vi "Pre-Build Action.vi"(6 "Top Level/Always Included VIs":path[](array[path]), 7 "Main Destination Path":path, 9 "Target Name":string, 10 "Build Specification Name":string, 11 "Project Path":path) -> (0 "error out":errorcluster)   [LabVIEW 2026]
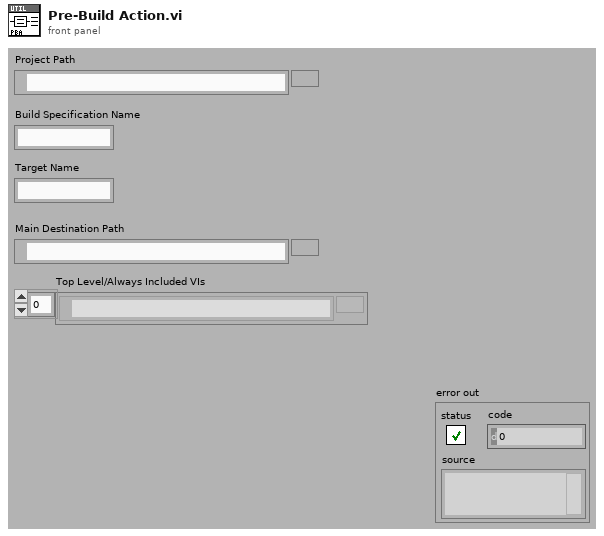
[diagram p1: front panel]
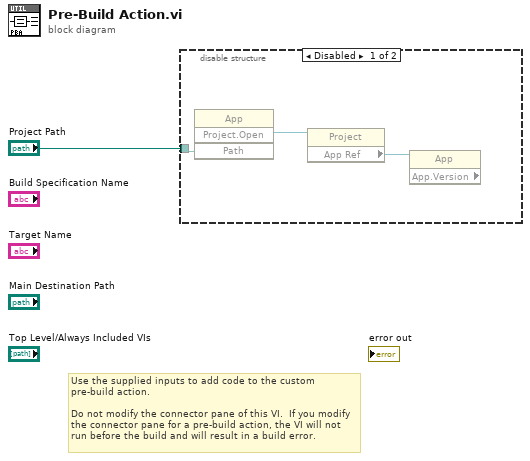
[diagram p0: block diagram]
diagram:
  # "Use the supplied inputs to add code to the custom pre-build action.\n\nDo not modify the connector pane of this VI.  If you modify the connector pane for a pre-build action, the VI will not run before the build and will result in a build error."
  n1 = disable-structure shown="Disabled" {
    disable-tunnel: "Project Path" -> [w4 _]
    frame Disabled {
      n2 = invoke class="App" method="Project.Open"("Path"=w4) -> ("Project:Open"=w3:refnum<vi>)  [unwired: 3 in, 3 out]
      n3 = property class="Project"(reference=w3) -> ("App Ref"=w2:refnum<vi>)  [unwired: 1 in, 2 out]
      n4 = property class="App" props=["App.Version"](reference=w2) -> ()  [unwired: 1 in, 3 out]
    }
    frame Enabled {
    }
  }
